vi "XY Graph Straighten Decay [Core] v3.vi"(8 "Error In":errorcluster, 9 "End index (-1: Last)":i32=-1, 10 "Start index (0: First)":i32, 11 "Plot in":cluster{"X Array":dbl[], "Y Array":dbl[]}) -> (0 "error out":errorcluster, 1 "Fitted Tau":dbl, 3 "Plot out":cluster{"X Array":dbl[], "Y Array":dbl[]})   [LabVIEW 2021, in "XY Graph Add-Ons.lvlib"]
doc: "Corrects a single period of a periodic decay, when the decay starts at the first data point and ends at the last point, in the presence of a single-exponential damping (due for instance to fluorescence photobleaching).\n\nThe correction is in general still valid when the last provided point is not exactly the period."
uses:
  XY Graph Add-Ons.lvlib
  <vilib>/Utility/error.llb/Error Cluster From Error Code.vi
  <vilib>/ErrorRing/Error Ring.xnode
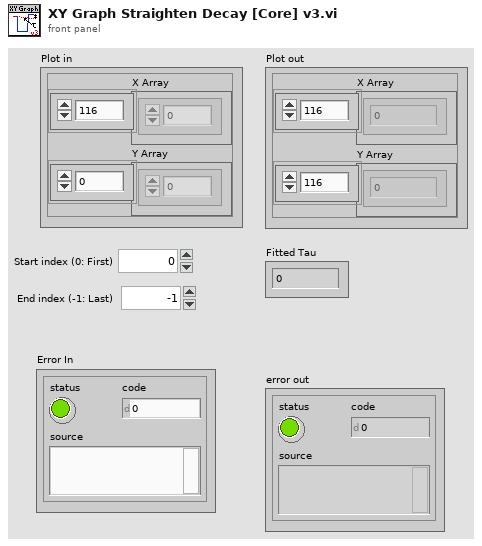
[diagram p1: front panel]
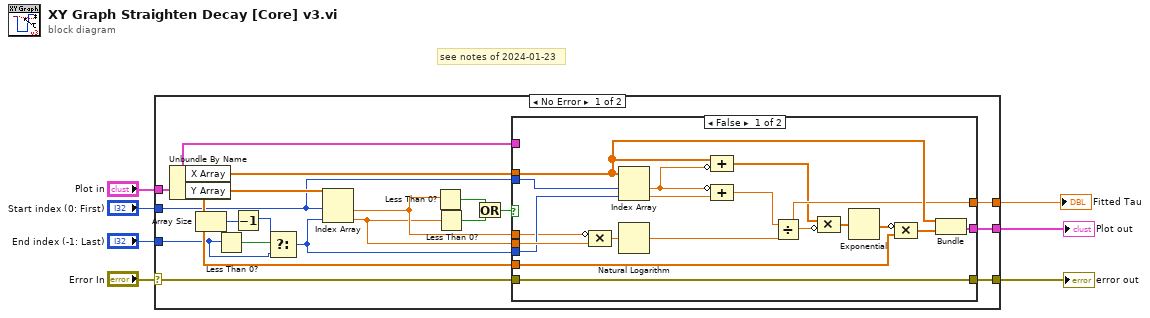
[diagram p0: block diagram]
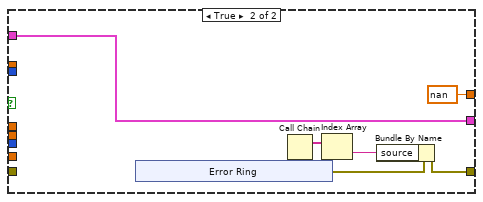
[diagram p2: hidden frame]
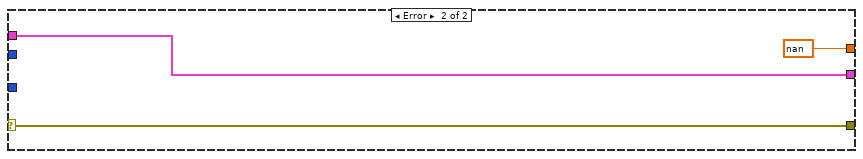
[diagram p3: hidden frame]
diagram:
  # "see notes of 2024-01-23"
  n1 = case shown="No Error" "Error In" {
    selector: "Error In" -> [w15 w56]
    tunnel: "Plot in" -> [w16 w55]
    tunnel: [w14 w56] -> w5
    tunnel: [w23 w55] -> w4
    tunnel: [w22 nan] -> w3
    tunnel: "Start index (0: First)" -> [w9 _]
    tunnel: "End index (-1: Last)" -> [w10 _]
    frame No Error {
      n2 = Unbundle By Name(w16) -> ("X Array"=w24:dbl[], "Y Array"=w18:dbl[])
      n3 = Array Size(array=w18) -> (size(s)=w25:i32)
      n4 = Less Than 0?(x=w10) -> (x < 0?=w12:bool)
      n5 = Decrement(x=w25) -> (x-1=w11:i32)
      n6 = Select(t=w11, s=w12, f=w10) -> (s? t:f=w8:i32)
      n7 = Index Array(array=w18, index #1=w9, index #2=w8) -> (element #1=w19:dbl, element #2=w13:dbl)
      n8 = Less Than 0?(x=w19) -> (x < 0?=w21:bool)
      n9 = Less Than 0?(x=w13) -> (x < 0?=w20:bool)
      n10 = Or(x=w21, y=w20) -> (x .or. y?=w17:bool)
      n11 = case shown="False" w17 {
        tunnel: w13 -> [w43 _]
        tunnel: w24 -> [w42 _]
        tunnel: w8 -> [w41 _]
        tunnel: [w40 w49] -> w23
        tunnel: [w39 nan] -> w22
        tunnel: w19 -> [w30 _]
        tunnel: w18 -> [w29 _]
        tunnel: w16 -> [_ w49]
        tunnel: w15 -> [w27 _]
        tunnel: [w27 w46] -> w14
        tunnel: w9 -> [w26 _]
        frame False {
          n12 = Compound Arithmetic op=MULTIPLY(invert w30, w43) -> (w38:dbl)
          n13 = Index Array(array=w42, index #1=w26, index #2=w41) -> (element #1=w36:dbl, element #2=w37:dbl)
          n14 = Natural Logarithm(1:w38) -> (0:w33:dbl)
          n15 = Compound Arithmetic op=ADD(w42, invert w36) -> (w35:dbl[])
          n16 = Compound Arithmetic op=ADD(invert w36, w37) -> (w32:dbl)
          n17 = Divide(x=w32, y=w33) -> (x/y=w39:dbl)
          n18 = Compound Arithmetic op=MULTIPLY(w35, invert w39) -> (w34:dbl[])
          n19 = Exponential(1:w34) -> (0:w31:dbl[])
          n20 = Compound Arithmetic op=MULTIPLY(invert w31, w29) -> (w28:dbl[])
          n21 = Bundle("X Array"=w42, w28) -> (w40:cluster{"X Array":dbl[], dbl[]})  [unwired: 1 in]
        }
        frame True {
          n22 = xnode "Error Ring"() -> ("error out"=w47:errorcluster)
          n23 = Call Chain() -> (call chain=w45:string[])
          n24 = Index Array(array=w45) -> (element=w44:string)  [unwired: 1 in]
          n25 = Bundle By Name(cluster=w47, "source"=w44) -> (w46:errorcluster)
        }
      }
    }
    frame Error {
    }
  }
  "error out" <- w5
  "Fitted Tau" <- w3
  "Plot out" <- w4
